vi "ConnectionStateChanged Event Callback.vi"(4 "User Parameter":refnum<user-event>, 5 "Event Data":cluster{"sender":refnum<k24>, "e":refnum<k24>}, 6 "Control Ref":refnum<k24>, 7 "Event Common Data":T1) -> ()   [LabVIEW 2018, in "TwinCAT ADS.lvclass"]
uses:
  TwinCAT ADS.lvclass
  TwinCAT.Ads
  Controls/Connection State Change Event Data.ctl
  <vilib>/event_ctls.llb/usereventprio.ctl
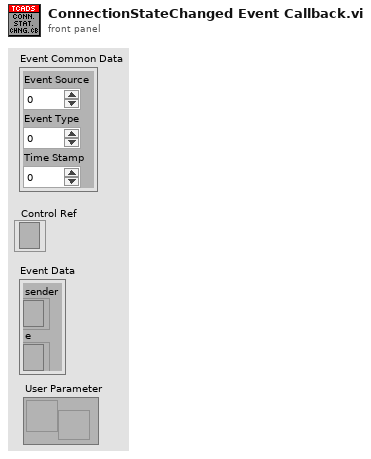
[diagram p1: front panel]
types:
  T1 = cluster{"Event Source":i32, "Event Type":u32, "Time Stamp":u32}
  T2 = typedef "usereventprio.ctl" = enum32{"high priority", "normal priority"}
  T3 = typedef "TwinCAT ADS.lvclass/Connection State Change Event Data.ctl" = cluster{"Old State":enum16{"None, Unknown", "Disconnected", "Connected", "Lost"}, "New State":enum16{"None, Unknown", "Disconnected", "Connected", "Lost"}, "Reason":enum16{"None", "Established", "Closed", "Lost", "Error", "Resurrected"}}
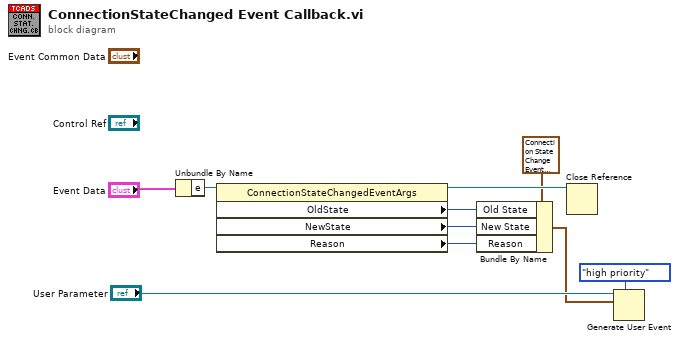
[diagram p0: block diagram]
diagram:
  n1 = Unbundle By Name("Event Data") -> ("e"=w8:refnum<k24>)
  n2 = property class="ConnectionStateChangedEventArgs"(reference=w8) -> (reference out=w10:refnum<k24>, "OldState"=w4:i32, "NewState"=w5:i32, "Reason"=w6:i32)  [unwired: 1 in, 1 out]
  n3 = Bundle By Name(cluster=T3 {"Old State"=enum."None, Unknown", "New State"=enum."None, Unknown", "Reason"=enum."None"} ("Connection State Change Event Data"), "Old State"=w4, "New State"=w5, "Reason"=w6) -> (w2:T3)
  n4 = Close Reference(reference=w10) -> ()  [unwired: 1 in, 1 out]
  n5 = Generate User Event(priority (normal)=usereventprio."high priority", user event="User Parameter", event data cluster=w2) -> ()  [unwired: 1 in, 2 out]
